vi "VAT_valve_set_operating_mode.vi"(0 "VAT Valve COM port":refnum<visa-resource-name>, 2 "Operating Mode":u16(ring) items=["Pressure", "Flow", "Stop"], 11 "error in (no error)":errorcluster) -> (4 "VAT Valve COM port out":refnum<visa-resource-name>, 15 "error out":errorcluster)   [LabVIEW 2019]
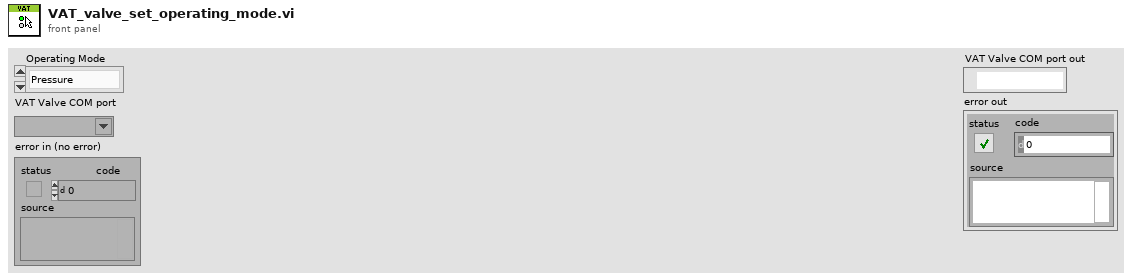
[diagram p1: front panel]
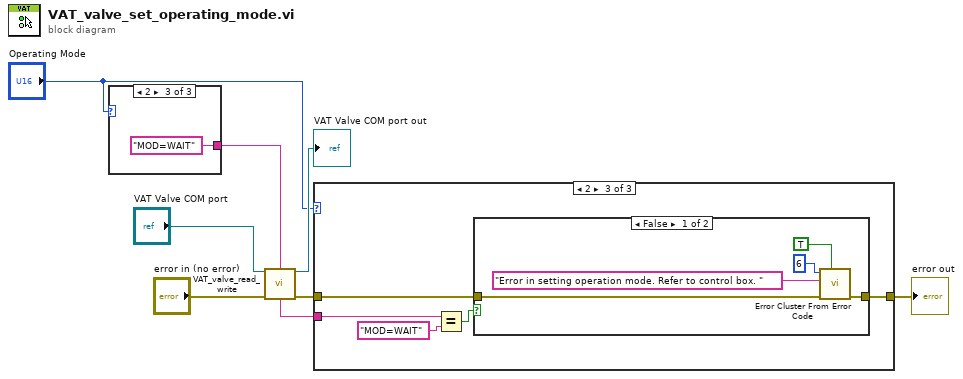
[diagram p0: block diagram]
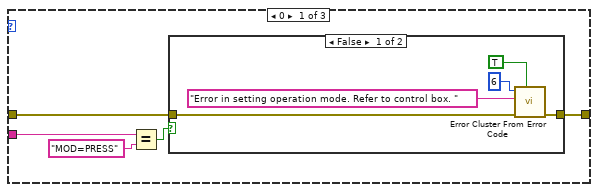
[diagram p2: hidden frame]
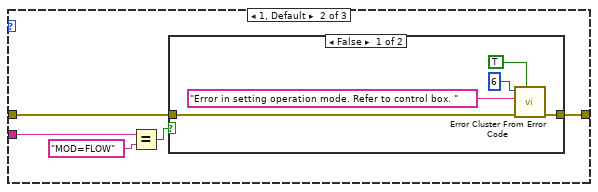
[diagram p4: hidden frame]
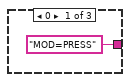
[diagram p7: hidden frame]
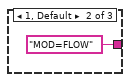
[diagram p8: hidden frame]
diagram:
  n1 = case shown="2" "Operating Mode" {
    tunnel: ["MOD=PRESS" "MOD=FLOW" "MOD=WAIT"] -> w8
    frame 0 {
    }
    frame 1, Default {
    }
    frame 2 {
    }
  }
  n2 = call "VAT_valve_read_write.vi"("VAT Valve COM port"="VAT Valve COM port", "Write String"=w8, "error in (no error)"="error in (no error)") -> ("VAT Valve COM port out"=→"VAT Valve COM port out":refnum<visa-resource-name>, "Read String"=w3:string, "error out"=w2:errorcluster)  [unwired: 10 in]
  n3 = case shown="2" "Operating Mode" {
    tunnel: w3 -> [w16 w27 w38]
    tunnel: w2 -> [w13 w24 w35]
    tunnel: [w12 w23 w34] -> w1
    frame 0 {
      n4 = Equal?(x=w16, y="MOD=PRESS") -> (x = y?=w14:bool)
      n5 = case shown="False" w14 {
        tunnel: w13 -> [w20 w22]
        tunnel: [w21 w22] -> w12
        frame False {
          n6 = call <vilib>:"Error Cluster From Error Code.vi"("show call chain? (False)"=TRUE, "error in (no error)"=w20, "error message (\"\")"="Error in setting operation mode. Refer to control box. " ("error message (\"\")"), "error code (0)"=6) -> ("error out"=w21:errorcluster)  [unwired: 5 in]
        }
        frame True {
        }
      }
    }
    frame 1, Default {
      n7 = Equal?(x=w27, y="MOD=FLOW") -> (x = y?=w25:bool)
      n8 = case shown="False" w25 {
        tunnel: w24 -> [w31 w33]
        tunnel: [w32 w33] -> w23
        frame False {
          n9 = call <vilib>:"Error Cluster From Error Code.vi"("show call chain? (False)"=TRUE, "error in (no error)"=w31, "error message (\"\")"="Error in setting operation mode. Refer to control box. " ("error message (\"\")"), "error code (0)"=6) -> ("error out"=w32:errorcluster)  [unwired: 5 in]
        }
        frame True {
        }
      }
    }
    frame 2 {
      n10 = Equal?(x=w38, y="MOD=WAIT") -> (x = y?=w36:bool)
      n11 = case shown="False" w36 {
        tunnel: w35 -> [w42 w44]
        tunnel: [w43 w44] -> w34
        frame False {
          n12 = call <vilib>:"Error Cluster From Error Code.vi"("show call chain? (False)"=TRUE, "error in (no error)"=w42, "error message (\"\")"="Error in setting operation mode. Refer to control box. " ("error message (\"\")"), "error code (0)"=6) -> ("error out"=w43:errorcluster)  [unwired: 5 in]
        }
        frame True {
        }
      }
    }
  }
  "error out" <- w1
